vi "Process.vi"(8 "error in":errorcluster, 11 "Inst.AH2500":refnum<class "Inst.AH2500.lvclass">) -> (0 "error out":errorcluster, 3 "Inst.AH2500 out":refnum<class "Inst.AH2500.lvclass">)   [LabVIEW 2019, in "Inst.AH2500.lvclass"]
doc: "---------------------------------------------------------------\nJKI State Machine Objects™\nhttp://jki.net/state-machine-objects/\nCopyright (C) 2005-2015, JKI <info@jki.net>\nALL RIGHTS RESERVED"
uses:
  Inst.AH2500.lvclass
  <vilib>/JKI/JKI SMO/SMO/SMO.lvclass
  <userlib>/LevyLab/Instrument Framework/Instrument/Instrument.lvclass
  <userlib>/LevyLab/RemoteControl/RemoteControl/Typedefs/Message--Cluster.ctl
  <userlib>/LevyLab/RemoteControl/RemoteControl/RemoteControl.lvclass
  Typedefs/PrivateEvents--Inst.AH2500.MessageToProcess.ctl
  C:/Program Files/National Instruments/LabVIEW 2019/user.lib/LevyLab/Instrument Framework/Instrument Types/CBridge/Instrument.CBridge.lvclass
  C:/Program Files/National Instruments/LabVIEW 2019/user.lib/LevyLab/Instrument Framework/Instrument/Instrument.lvclass
  C:/Program Files/National Instruments/LabVIEW 2019/vi.lib/JKI/JKI SMO/SMO/SMO.lvclass
  <userlib>/LevyLab/Instrument Framework/Instrument/API/Instrument.sendMessageToProcess (variant).vi
  <userlib>/LevyLab/Debug/Debug.lvlib
  <userlib>/LevyLab/Instrument Framework/Instrument Types/CBridge/Instrument.CBridge.lvclass
panel:
  out "Status":string
  out "State History":string
  # "Inst.AH2500"
  # "Inst.AH2500"
  # "For instructions on how to use the JKI State Machine Objects, examples and video tutorials, visit:\nhttp://jki.net/state-machine-objects/\n\nJKI State Machine Objects™\nhttp://jki.net/state-machine-objects/\nCopyright (C) 2005-2015, JKI <info@jki.net>\nALL RIGHTS RESERVED"
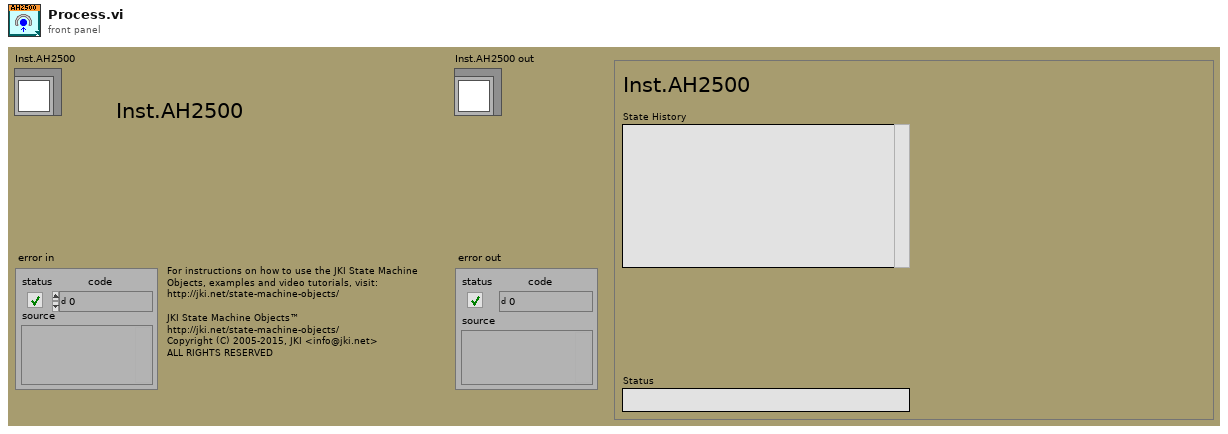
[diagram p1: front panel]
types:
  T1 = enum32{"invalid app kind", "Development System", "Run Time System", "Student Edition", "Embedded LabVIEW", "Evaluation", "Custom"}
  T2 = enum32{"Invalid", "Standard", "Closed", "Hidden", "Minimized", "Maximized"}
  T3 = typedef "RemoteControl.lvlib/RemoteControl.lvclass/Message--Cluster.ctl" = cluster{"Command":string, "Data":variant, "ID":string, "error":errorcluster}
  T4 = typedef "Inst.AH2500.lvclass/PrivateEvents--Inst.AH2500.MessageToProcess.ctl" = cluster{"Message":T3}
  T5 = cluster{"Core":cluster{"Current VI Reference":refnum<vi>, "Close Panel on Exit?":bool, "Last Error":cluster{"error":errorcluster, "previous state":string, "remaining states":string}, "Shutdown?":bool}, "SMO":refnum<class "Inst.AH2500.lvclass">, "Running Step":i32, "sequence":string[], "MessageToProcess":T4}
  T6 = cluster{"Current VI Reference":refnum<vi>, "Close Panel on Exit?":bool, "Last Error":cluster{"error":errorcluster, "previous state":string, "remaining states":string}, "Shutdown?":bool}
  T7 = typedef "Debug.lvlib/Attribute.Debug.lvclass/DebugBehavior.ctl" = enum16{"Normal", "Debug"}
  T8 = typedef "SMO.lvclass/Protected Events.ctl" = cluster{"StopProcesses":refnum<user-event>, "AbortProcesses":refnum<user-event>, "Config Changed":refnum<user-event>, "Dependency":refnum<user-event>}
  T9 = typedef "Inst.AH2500.lvclass/Inst.AH2500.getAll--Cluster.ctl" = cluster{"capacitance (pF)":dbl, "loss (nS)":dbl, "Vexc (V)":dbl}
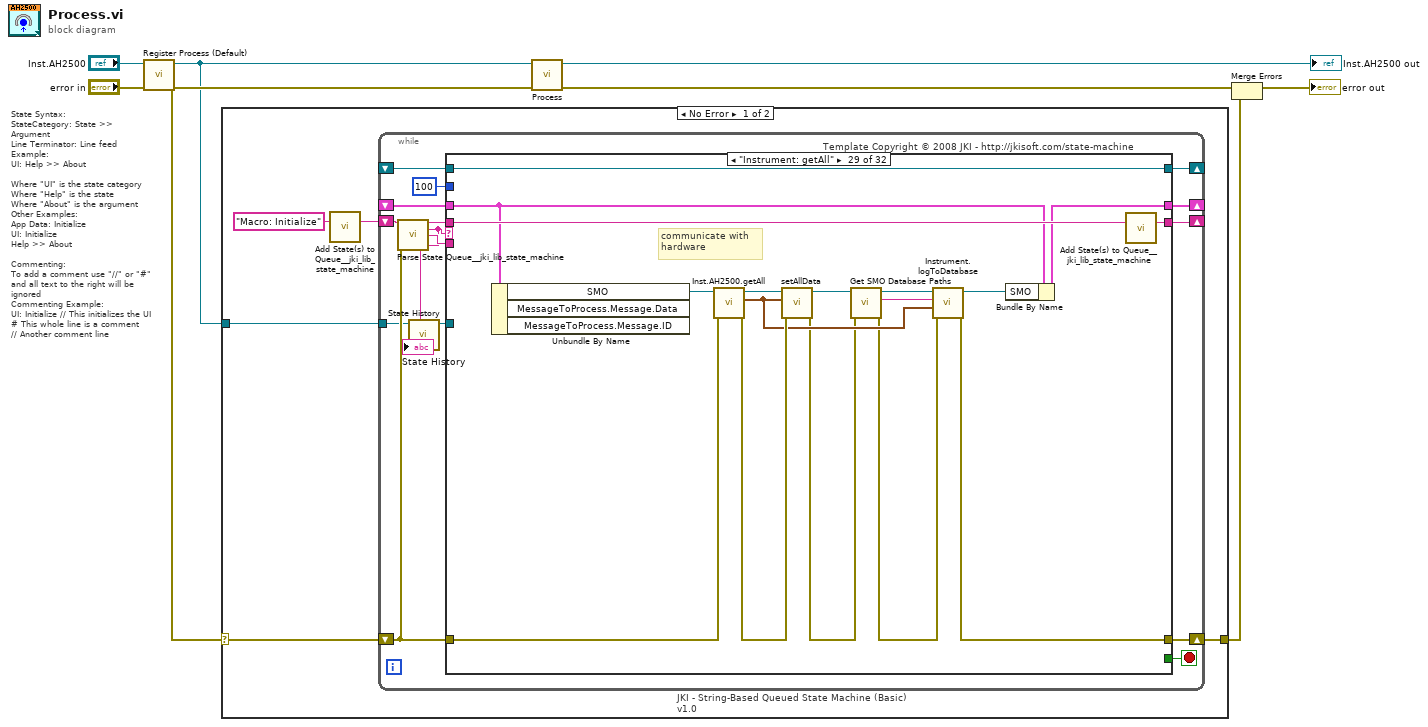
[diagram p0: block diagram]
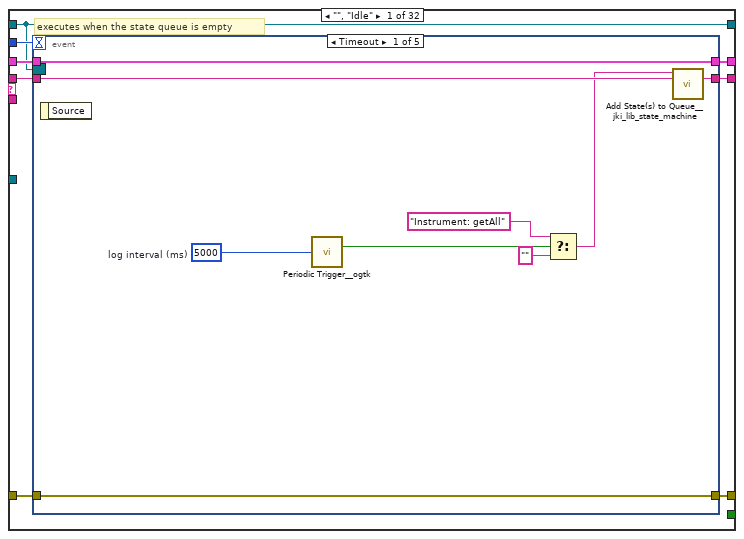
[diagram p2: hidden frame]
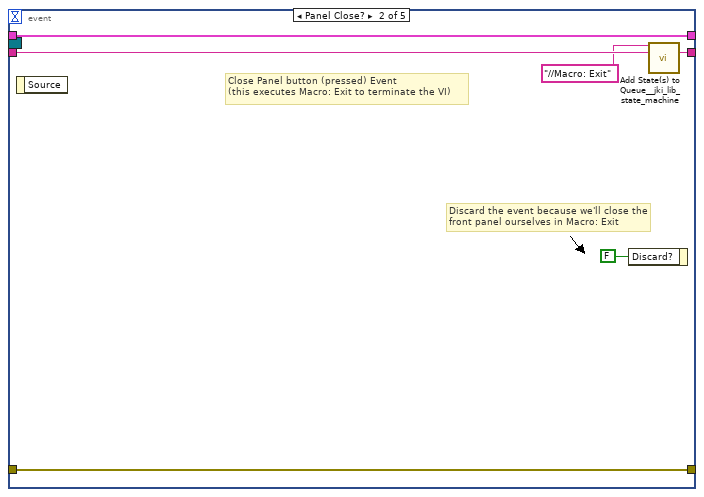
[diagram p3: hidden frame]
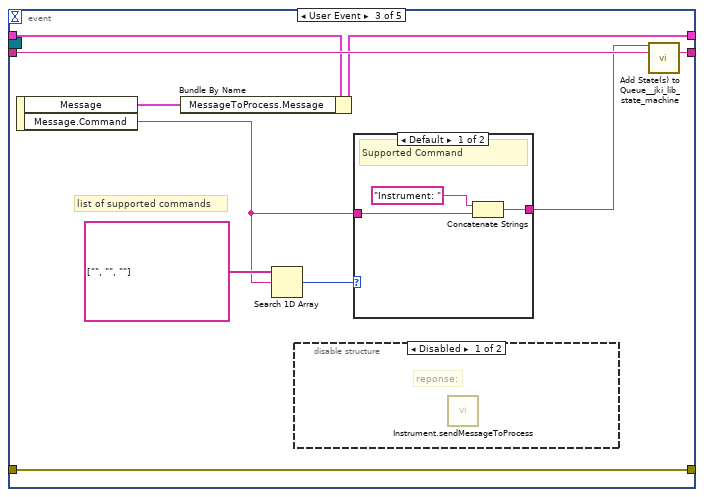
[diagram p4: hidden frame]
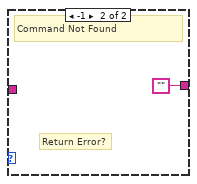
[diagram p6: hidden frame]
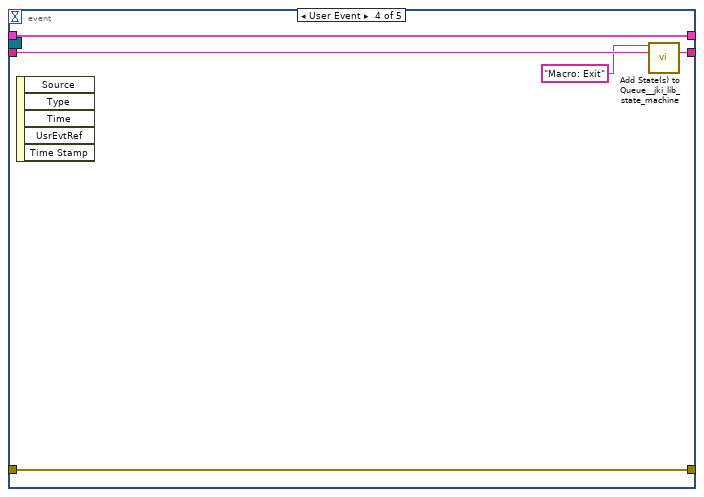
[diagram p7: hidden frame]
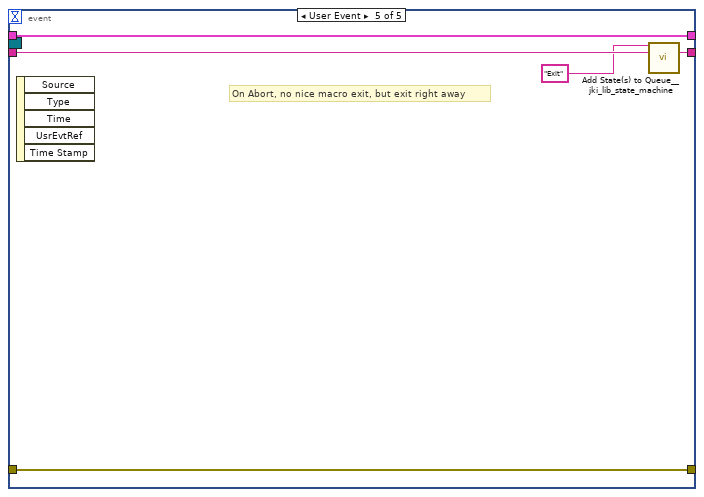
[diagram p8: hidden frame]
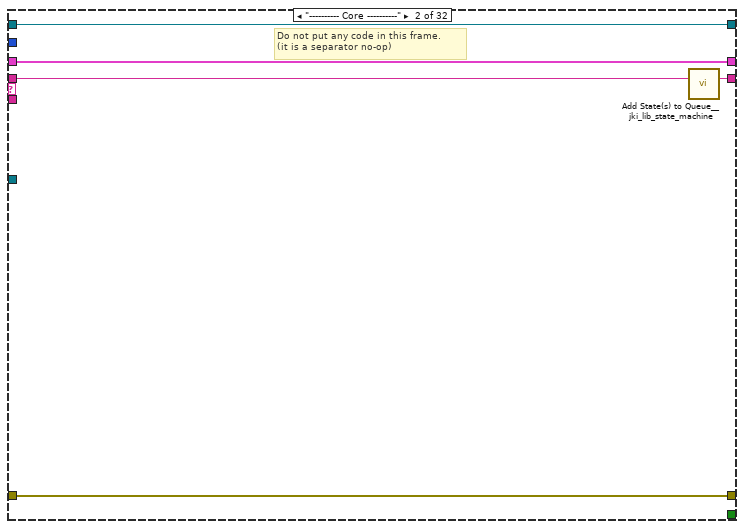
[diagram p9: hidden frame]
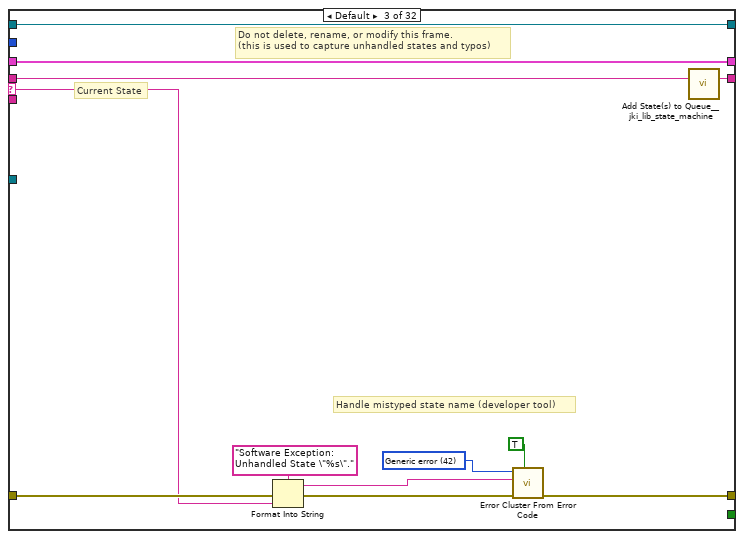
[diagram p10: hidden frame]
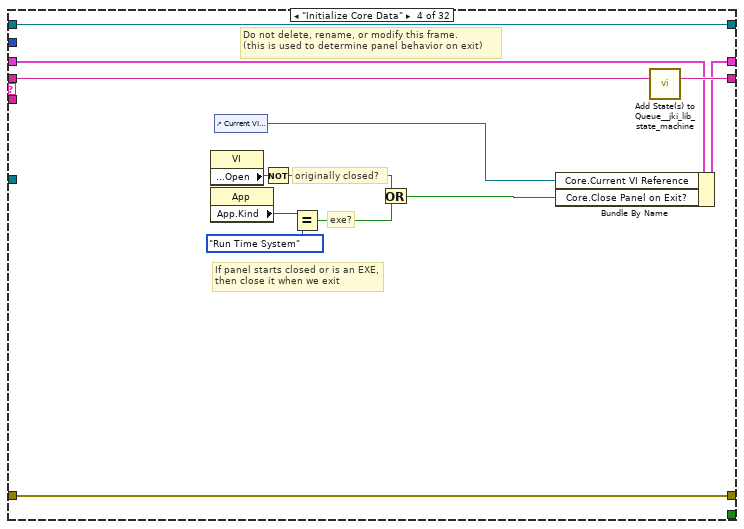
[diagram p11: hidden frame]
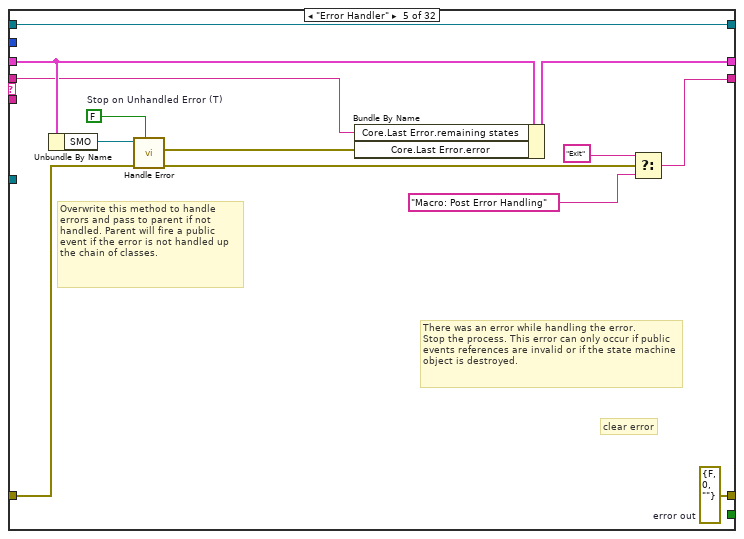
[diagram p12: hidden frame]
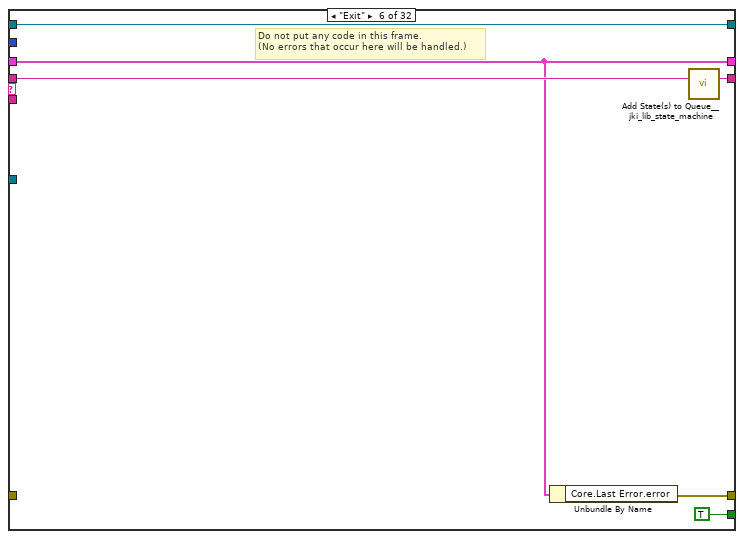
[diagram p13: hidden frame]
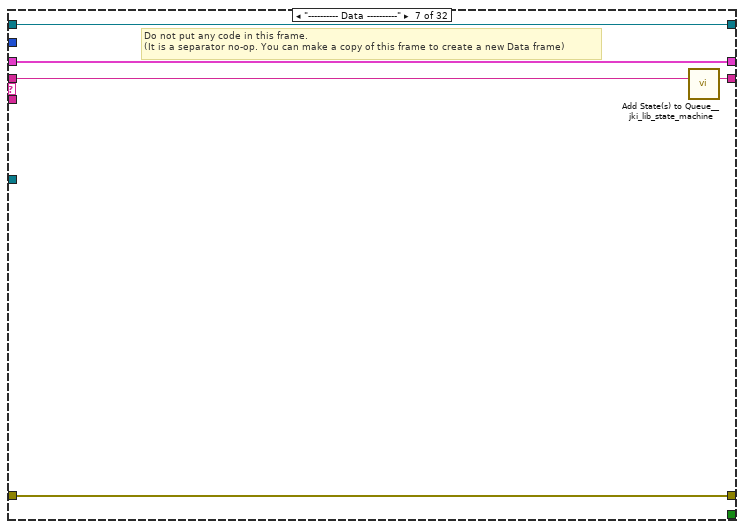
[diagram p14: hidden frame]
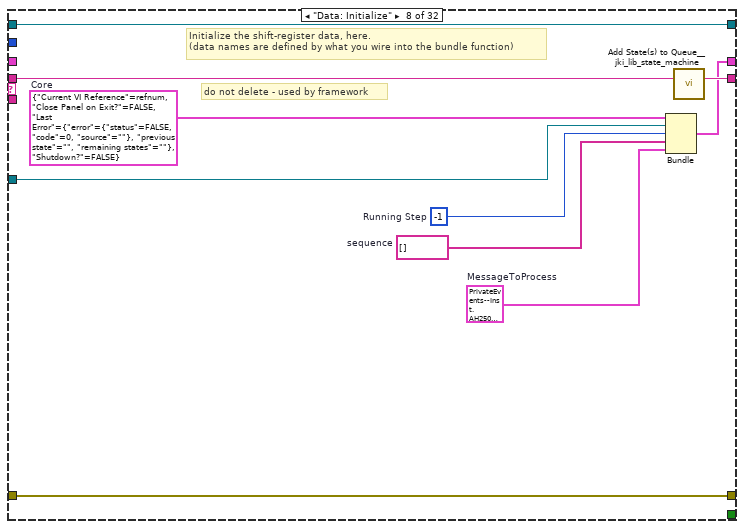
[diagram p15: hidden frame]
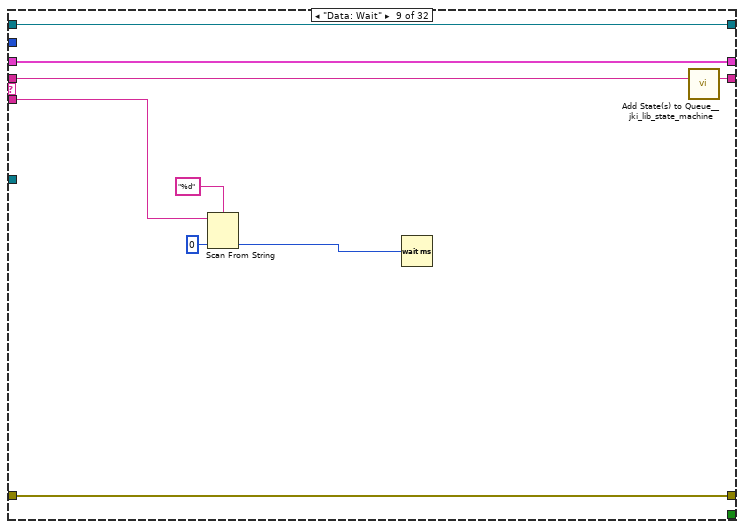
[diagram p16: hidden frame]
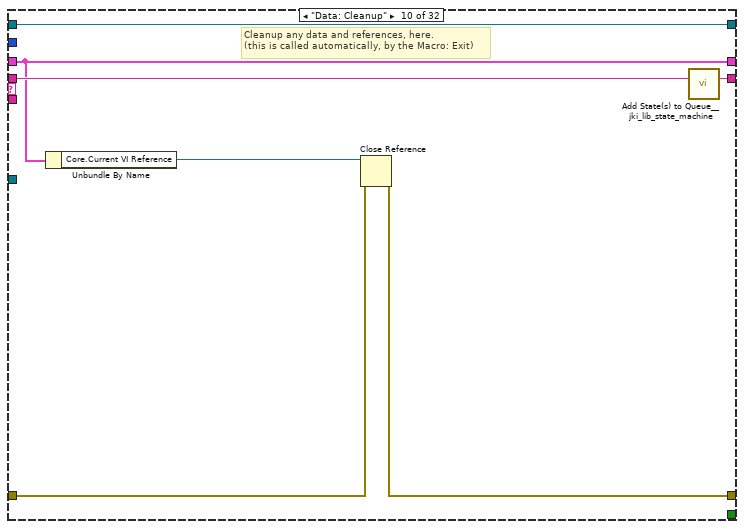
[diagram p17: hidden frame]
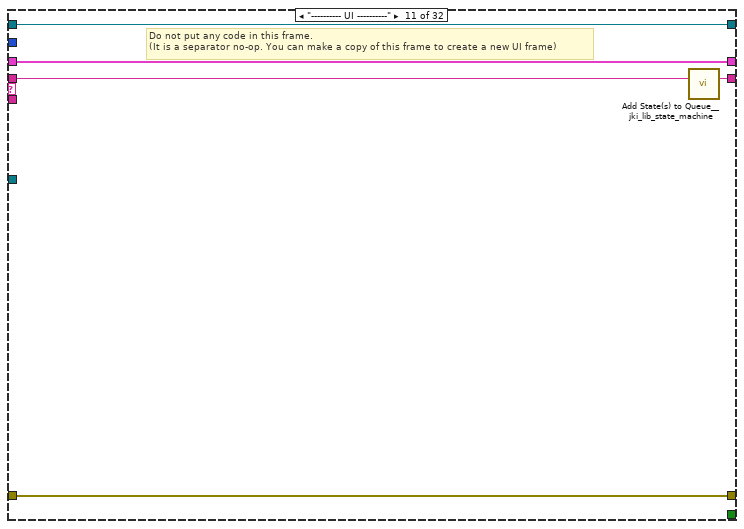
[diagram p18: hidden frame]
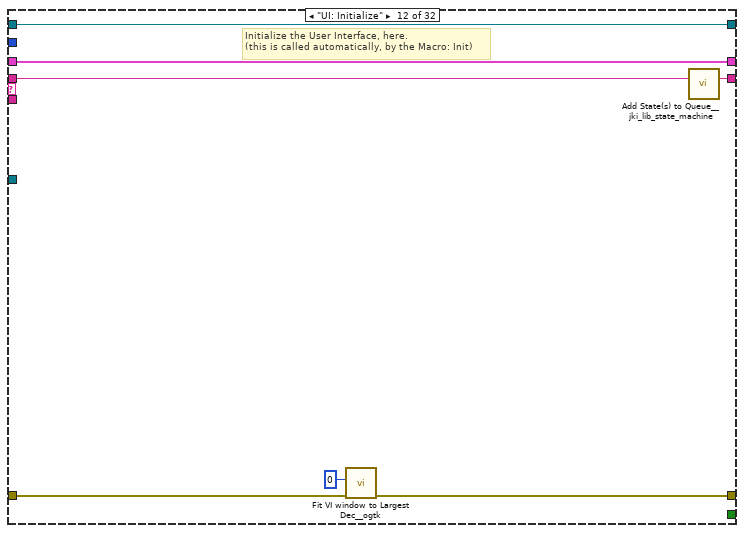
[diagram p19: hidden frame]
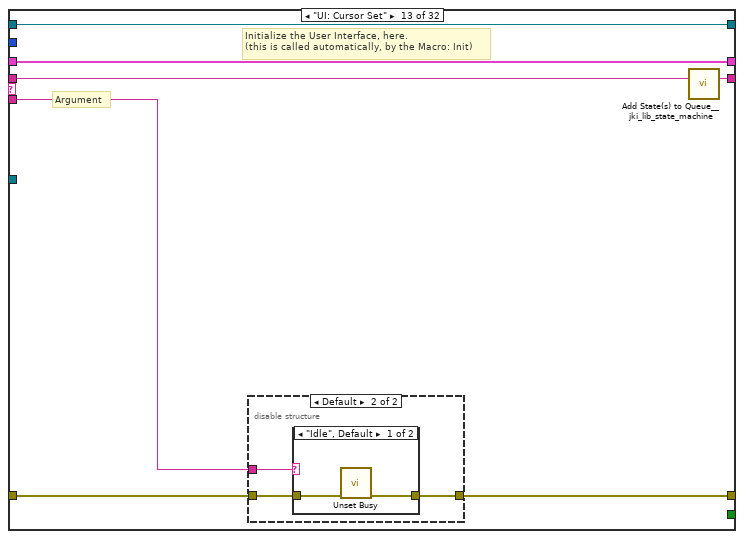
[diagram p20: hidden frame]
diagram:
  # "State Syntax:\nStateCategory: State >> Argument\nLine Terminator: Line feed\nExample:\nUI: Help >> About\n\nWhere \"UI\" is the state category\nWhere \"Help\" is the state\nWhere \"About\" is the argument\nOther Examples:\nApp Data: Initialize\nUI: Initialize\nHelp >> About\n\nCommenting:\nTo add a comment use \"//\" or \"#\" and all text to the right will be ignored\nCommenting Example:\nUI: Initialize // This initializes the UI\n# This whole line is a comment\n// Another comment line"
  n1 = call <vilib>:"Register Process (Default).vi"("error in (no error)"="error in", "SMO"="Inst.AH2500") -> ("error out"=w5:errorcluster, "SelfRef"=w4:refnum<class "Inst.AH2500.lvclass">)  [unwired: 8 in]
  n2 = case shown="No Error" w5 {
    selector: w5 -> [w10 w416]
    tunnel: w4 -> [w11 _]
    tunnel: [w9 w416] -> w1
    frame No Error {
      n3 = call <vilib>:"Add State(s) to Queue__jki_lib_state_machine.vi"("State(s) in (\"\")"="Macro: Initialize") -> ("States Out"=w13:string)  [unwired: 14 in]
      n4 = while "JKI - String-Based Queued State Machine (Basic) v1.0" {
        shift-right: [w23] -> _
        shift-left: _ -> [w22]
        shift-right: [w26] -> w9
        shift-left: w10 -> [w20]
        shift-right: [w25] -> _
        shift-left: w13 -> [w27]
        tunnel: w11 -> [w14]
        shift-right: [w19] -> _
        shift-left: _ -> [w18]
        stop <- w24 stop-if-true
        # "Template Copyright © 2008 JKI - http://jkisoft.com/state-machine"
        n5 = call <vilib>:"Parse State Queue__jki_lib_state_machine.vi"("State Queue"=w27, "Error In (no error)"=w20) -> ("Remaining States"=w29:string, "Current State"=w17:string, "Arguments"=w28:string)  [unwired: 11 in]
        n6 = call <userlib>:"State History.vi"("Current State"=w17, "SMO"=w14) -> ("SMO"=w15:refnum<class "Inst.AH2500.lvclass">, "History"=→"State History":string)  [unwired: 8 in]
        n7 = case shown="\"Instrument: getAll\"" w17 {
          selector: w17 -> [_ _ w83 _ _ _ _ _ _ _ _ _ _ _ _ _ _ _ _ _ _ _ _ _ _ _ _ _ _ _ _ _]
          tunnel: w29 -> [w37 w81 w87 w106 w111 w125 w130 w140 w149 w156 w161 w168 w175 w191 w223 w232 w236 w265 w286 w303 w308 w319 w324 w337 w343 w350 w359 w368 w385 w390 w396 w415]
          tunnel: w28 -> [_ _ _ _ _ _ _ _ w141 _ _ _ w169 w185 _ _ _ _ _ _ _ _ _ _ _ _ _ _ _ _ w391 w399]
          tunnel: w22 -> [w35 w78 w85 w97 w115 w121 w127 _ w146 w151 w158 w166 w173 w187 w220 w229 w235 w255 w276 w289 w305 w316 w321 w330 w341 w345 w355 w364 w381 w386 w392 w405]
          tunnel: [w34 w79 w89 w103 w116 w120 w128 w132 w147 w152 w159 w163 w170 w188 w221 w224 w239 w263 w284 w287 w306 w310 w322 w333 w339 w347 w352 w361 w369 w387 w393 w407] -> w26
          tunnel: w20 -> [w33 w79 w88 w103 w117 _ w128 w132 w147 w153 w159 w162 w171 w189 w221 w224 w238 w263 w284 w287 w306 w311 w322 w327 w339 w347 w351 w360 w379 w387 w393 w401]
          tunnel: [w36 w80 w86 w105 w107 w124 w129 w139 w148 w155 w160 w167 w174 w190 w222 w231 w234 w264 w285 w302 w307 w318 w323 w336 w342 w349 w358 w367 w384 w389 w395 w414] -> w25
          tunnel: [_ _ _ _ _ TRUE _ _ _ _ _ _ _ _ _ _ _ _ _ _ _ _ _ _ _ _ _ _ _ _ _ _] -> w24
          tunnel: [w32 w78 w85 w104 w114 w121 w127 w138 w146 w151 w158 w166 w173 w187 w220 w229 w237 w256 w277 w290 w305 w316 w321 w330 w341 w346 w356 w365 w382 w386 w392 w404] -> w23
          tunnel: 100 ("Timeout") -> [w31 _ _ _ _ _ _ _ _ _ _ _ _ _ _ _ _ _ _ _ _ _ _ _ _ _ _ _ _ _ _ _]
          tunnel: w15 -> [_ _ _ _ _ _ _ w133 _ _ _ _ _ _ _ _ _ _ _ _ _ _ _ _ _ _ _ _ _ _ _ _]
          tunnel: [w30 w77 w82 w94 w119 w122 w126 w137 w145 w150 w157 w165 w172 w184 w219 w230 w247 w262 w283 w297 w304 w317 w320 w335 w340 w348 w357 w366 w383 w388 w394 w413] -> w19
          tunnel: w18 -> [w30 w77 w82 w94 w119 w122 w126 w137 w145 w150 w157 w165 w172 w184 w219 w230 w247 w262 w283 w297 w304 w317 w320 _ w340 w348 w357 w366 w383 w388 w394 w413]
          frame "", "Idle" {
            # "executes when the state queue is empty"
            n8 = event shown="[0] Timeout" {
              selector: w30 -> [_ _ _ _ _]
              dyn-events: _ -> [_ _ _ _ _]
              timeout: w31 -> [_ _ _ _ _]
              tunnel: w37 -> [w46 w52 w62 w71 w76]
              tunnel: [w45 w51 w61 w70 w75] -> w36
              tunnel: w35 -> [w43 w49 w54 w68 w73]
              tunnel: [w44 w50 w60 w69 w74] -> w34
              tunnel: w33 -> [w44 w50 w60 w69 w74]
              tunnel: [w43 w49 w55 w68 w73] -> w32
              event Timeout {
                w40 = u32 5000  # log interval (ms)
                n9 = event-data() -> ()  [unwired: 1 in, 1 out]
                n10 = call <userlib>:"Periodic Trigger__ogtk.vi"("time (ms)"=w40) -> ("Triggered"=w42:bool)  [unwired: 12 in, 2 out]
                n11 = Select(t="Instrument: getAll", s=w42, f="") -> (s? t:f=w39:string)
                n12 = call <vilib>:"Add State(s) to Queue__jki_lib_state_machine.vi"("State(s) in Front (\"\")"=w39, "State(s) in (\"\")"=w46) -> ("States Out"=w45:string)  [unwired: 13 in]
              }
              event Panel Close? {
                # "Discard the event because we'll close the front panel ourselves in Macro: Exit"
                # "Close Panel button (pressed) Event\n(this executes Macro: Exit to terminate the VI)"
                n13 = event-data() -> ()  [unwired: 1 in, 1 out]
                n14 = event-data("Discard?"=FALSE) -> ()  [unwired: 1 in, 1 out]
                n15 = call <vilib>:"Add State(s) to Queue__jki_lib_state_machine.vi"("State(s) in Front (\"\")"="//Macro: Exit", "State(s) in (\"\")"=w52) -> ("States Out"=w51:string)  [unwired: 13 in]
              }
              event User Event {
                # "list of supported commands"
                n16 = event-data() -> ("Message"=w53:T3, "Message.Command"=w56:string)  [unwired: 1 in]
                n17 = Bundle By Name(cluster=w54, "MessageToProcess.Message"=w53) -> (w55:T5)
                n18 = Search 1D Array(1D array=string[] ["", "", ""], element=w56) -> (index of element=w59:i32)  [unwired: 1 in]
                n19 = disable-structure shown="Disabled" {
                  frame Disabled {
                    # "reponse:"
                    n20 = call-poly <userlib>:"Instrument.sendMessageToProcess.vi"() -> ()  [unwired: 10 in, 2 out]
                  }
                  frame Enabled {
                  }
                }
                n21 = case shown="Default" w59 {
                  tunnel: [w65 "" ("Empty String Constant")] -> w57
                  tunnel: w56 -> [w64 _]
                  frame Default {
                    # "Supported Command"
                    n22 = Concatenate Strings("Instrument: ", w64) -> (w65:string)
                  }
                  frame -1 {
                    # "Return Error?"
                    # "Command Not Found"
                  }
                }
                n23 = call <vilib>:"Add State(s) to Queue__jki_lib_state_machine.vi"("State(s) in Front (\"\")"=w57, "State(s) in (\"\")"=w62) -> ("States Out"=w61:string)  [unwired: 13 in]
              }
              event User Event {
                n24 = event-data() -> ()  [unwired: 1 in, 5 out]
                n25 = call <vilib>:"Add State(s) to Queue__jki_lib_state_machine.vi"("State(s) in Front (\"\")"="Macro: Exit", "State(s) in (\"\")"=w71) -> ("States Out"=w70:string)  [unwired: 13 in]
              }
              event User Event {
                # "On Abort, no nice macro exit, but exit right away"
                n26 = event-data() -> ()  [unwired: 1 in, 5 out]
                n27 = call <vilib>:"Add State(s) to Queue__jki_lib_state_machine.vi"("State(s) in Front (\"\")"="Exit", "State(s) in (\"\")"=w76) -> ("States Out"=w75:string)  [unwired: 13 in]
              }
            }
          }
          frame "---------- Core ----------" {
            # "Do not put any code in this frame.\n(it is a separator no-op)"
            n28 = call <vilib>:"Add State(s) to Queue__jki_lib_state_machine.vi"("State(s) in (\"\")"=w81) -> ("States Out"=w80:string)  [unwired: 14 in]
          }
          frame Default {
            w92 = 42 items=["No error", "Argument error", "Memory is full", "Out of zone", "End of file", "File already open", "Generic file I/O error", "File not found", "File permission error", "Disk is full", "Duplicate path", "Too many files open", "System feature not enabled", "Resource file not found", "Cannot add resource", "Resource not found", "Image not found", "Image memory error", "Pen does not exist", "Config type invalid", "Config token not found", "Config parse error", "Config memory error", "Bad external code format", "Bad external code offset", "External code not present", "Null window", "Destroy window error", "Null menu", "Print aborted", "Bad print record", "Print driver error", "Windows error during printing", "Memory error during printing", "Print dialog error", "Generic print error", "Invalid device refnum", "Device not found", "Device parameter error", "Device unit error", "Cannot open device", "Device call aborted", "Generic error", "Cancelled by user", "Object ID too low", "Object ID too high", "Object not in heap", "Unknown heap", "Unknown object (invalid DefProc)", "Unknown object (DefProc not in table)", "Message out of range", "Invalid (null) method", "Unknown message", "Manager call not supported", "Bad address", "Network operation in progress", "Network operation timed out", "Connection is busy", "Network attribute not supported", "Network error", "Address in use", "System out of memory", "Connection aborted", "Connection refused", "Not connected", "Already connected", "Connection closed", "Initialization error (interapplication manager)", "Bad occurrence", "Wait on unbound occurrence handler", "Occurrence queue overflow", "Datalog type conflict", "Unused", "Unrecognized type (interapplication manager)", "Memory corrupt", "Failed to make temporary DLL", "Old CIN version", "Drag socket not found", "Failed to load drop-object", "Failed to register OLE object", "Failed to release OLE object", "Format specifier type mismatch", "Unknown format specifier", "Too few format specifiers", "Too many format specifiers", "Scan failed", "Newer CIN version", "Error converting to variant", "Runtime menu error", "Password tampered", "Variant attribute not found", "Incompatible variant data type", "Event data is not available", "Event Store is not present", "Occurrence is not found", "Event Queue is not created", "Event info is not available", "Refnum passed is NULL", "Error retrieving Class GUID", "Error retrieving CoClass GUID", "Error retrieving TypeLib GUID.", "Bad built application magic bytes.", "Specific driver is different from the specific driver associated with the Logical Name.", "There is no session opened to the class driver.", "Max Error", "MAX - Error with config objects", "MAX - Error loading configuration", "MAX - Group not supported"]
            # "Current State"
            # "Do not delete, rename, or modify this frame.\n(this is used to capture unhandled states and typos)"
            # "Handle mistyped state name (developer tool)"
            n29 = Format Into String(format string="Software Exception: Unhandled State \"%s\"." ("message"), error in=w88, w83) -> (resulting string=w91:string, error out=w90:errorcluster)  [unwired: 1 in]
            n30 = call <vilib>:"Error Cluster From Error Code.vi"("show call chain? (False)"=TRUE, "error in (no error)"=w90, "error message (\"\")"=w91, "error code (0)"=w92) -> ("error out"=w89:errorcluster)  [unwired: 5 in]
            n31 = call <vilib>:"Add State(s) to Queue__jki_lib_state_machine.vi"("State(s) in (\"\")"=w87) -> ("States Out"=w86:string)  [unwired: 14 in]
          }
          frame "Initialize Core Data" {
            # "Do not delete, rename, or modify this frame.\n(this is used to determine panel behavior on exit)"
            # "originally closed?"
            # "exe?"
            # "If panel starts closed or is an EXE, then close it when we exit"
            n32 = property class="VI"() -> ("Front Panel.Open"=w102:bool)  [unwired: 2 in, 2 out]
            n33 = property class="App"() -> ("App.Kind"=w101:T1)  [unwired: 2 in, 2 out]
            n34 = control-ref of="Current VI Reference"() -> (w95:refnum<vi>)
            n35 = Not(x=w102) -> (.not. x?=w99:bool)
            n36 = Equal?(x=w101, y=T1."Run Time System" ("Application:Kind")) -> (x = y?=w98:bool)
            n37 = Or(x=w99, y=w98) -> (x .or. y?=w96:bool)
            n38 = Bundle By Name(cluster=w97, "Core.Current VI Reference"=w95, "Core.Close Panel on Exit?"=w96) -> (w104:T5)
            n39 = call <vilib>:"Add State(s) to Queue__jki_lib_state_machine.vi"("State(s) in (\"\")"=w106) -> ("States Out"=w105:string)  [unwired: 14 in]
          }
          frame "Error Handler" {
            w112 = FALSE  # Stop on Unhandled Error (T)
            w116 = errorcluster {"status"=FALSE, "code"=0, "source"=""}  # error out
            # "clear error"
            # "There was an error while handling the error.\nStop the process. This error can only occur if public events references are invalid or if the state machine object is destroyed."
            # "Overwrite this method to handle errors and pass to parent if not handled. Parent will fire a public event if the error is not handled up the chain of classes."
            n40 = Unbundle By Name(w115) -> ("SMO"=w118:refnum<class "Inst.AH2500.lvclass">)
            n41 = call-dynamic "Handle Error.vi"("Stop on Unhandled Error (T)"=w112, "error in"=w117, "SMO"=w118) -> ("handling error"=w108:errorcluster, "Unhandled error"=w113:errorcluster)  [unwired: 6 in, 1 out]
            n42 = Bundle By Name(cluster=w115, "Core.Last Error.remaining states"=w111, "Core.Last Error.error"=w113) -> (w114:T5)
            n43 = Select(t="Exit", s=w108, f="Macro: Post Error Handling") -> (s? t:f=w107:string)
          }
          frame "Exit" {
            # "Do not put any code in this frame.\n(No errors that occur here will be handled.)"
            n44 = Unbundle By Name(w121) -> ("Core.Last Error.error"=w120:errorcluster)
            n45 = call <vilib>:"Add State(s) to Queue__jki_lib_state_machine.vi"("State(s) in (\"\")"=w125) -> ("States Out"=w124:string)  [unwired: 14 in]
          }
          frame "---------- Data ----------" {
            # "Do not put any code in this frame.\n(It is a separator no-op. You can make a copy of this frame to create a new Data frame)"
            n46 = call <vilib>:"Add State(s) to Queue__jki_lib_state_machine.vi"("State(s) in (\"\")"=w130) -> ("States Out"=w129:string)  [unwired: 14 in]
          }
          frame "Data: Initialize" {
            w131 = T4 {"Message"={"Command"="", "Data"=variant(string ""), "ID"="", "error"={"status"=FALSE, "code"=0, "source"=""}}}  # MessageToProcess
            w134 = string[] []  # sequence
            w135 = -1  # Running Step
            w136 = T6 {"Current VI Reference"=refnum, "Close Panel on Exit?"=FALSE, "Last Error"={"error"={"status"=FALSE, "code"=0, "source"=""}, "previous state"="", "remaining states"=""}, "Shutdown?"=FALSE}  # Core
            # "do not delete - used by framework"
            # "Initialize the shift-register data, here.\n(data names are defined by what you wire into the bundle function)"
            n47 = Bundle("Core"=w136, "SMO"=w133, "Running Step"=w135, "sequence"=w134, "MessageToProcess"=w131) -> (w138:T5)  [unwired: 1 in]
            n48 = call <vilib>:"Add State(s) to Queue__jki_lib_state_machine.vi"("State(s) in (\"\")"=w140) -> ("States Out"=w139:string)  [unwired: 14 in]
          }
          frame "Data: Wait" {
            n49 = Scan From String(format string="%d", input string=w141, default 1=u32 0 ("default value 1")) -> (output 1=w142:u32)  [unwired: 2 in, 3 out]
            n50 = Wait (ms)(milliseconds to wait=w142) -> ()  [unwired: 1 out]
            n51 = call <vilib>:"Add State(s) to Queue__jki_lib_state_machine.vi"("State(s) in (\"\")"=w149) -> ("States Out"=w148:string)  [unwired: 14 in]
          }
          frame "Data: Cleanup" {
            # "Cleanup any data and references, here.\n(this is called automatically, by the Macro: Exit)"
            n52 = Unbundle By Name(w151) -> ("Core.Current VI Reference"=w154:refnum<vi>)
            n53 = Close Reference(reference=w154, error in (no error)=w153) -> (error out=w152:errorcluster)
            n54 = call <vilib>:"Add State(s) to Queue__jki_lib_state_machine.vi"("State(s) in (\"\")"=w156) -> ("States Out"=w155:string)  [unwired: 14 in]
          }
          frame "---------- UI ----------" {
            # "Do not put any code in this frame.\n(It is a separator no-op. You can make a copy of this frame to create a new UI frame)"
            n55 = call <vilib>:"Add State(s) to Queue__jki_lib_state_machine.vi"("State(s) in (\"\")"=w161) -> ("States Out"=w160:string)  [unwired: 14 in]
          }
          frame "UI: Initialize" {
            # "Initialize the User Interface, here.\n(this is called automatically, by the Macro: Init)"
            n56 = call <userlib>:"Fit VI window to Largest Dec__ogtk.vi"("error in (no error)"=w162, "border spacing (2 px)"=0) -> ("error out"=w163:errorcluster)  [unwired: 4 in, 1 out]
            n57 = call <vilib>:"Add State(s) to Queue__jki_lib_state_machine.vi"("State(s) in (\"\")"=w168) -> ("States Out"=w167:string)  [unwired: 14 in]
          }
          frame "UI: Cursor Set" {
            # "Argument"
            # "Initialize the User Interface, here.\n(this is called automatically, by the Macro: Init)"
            n58 = disable-structure shown="Default" {
              disable-tunnel: w171 -> [w176 w179]
              disable-tunnel: [w176 w178] -> w170
              disable-tunnel: w169 -> [_ w177]
              frame condition #0 {
              }
              frame condition #1 (active) {
                n59 = case shown="\"Idle\", Default" w177 {
                  tunnel: w179 -> [w181 w183]
                  tunnel: [w180 w182] -> w178
                  frame "Idle", Default {
                    n60 = call <vilib>:"Unset Busy.vi"("error in (no error)"=w181) -> ("error out"=w180:errorcluster)  [unwired: 10 in]
                  }
                  frame "Busy" {
                    n61 = call <vilib>:"Set Busy.vi"("error in (no error)"=w183) -> ("error out"=w182:errorcluster)  [unwired: 9 in, 1 out]
                  }
                }
              }
            }
            n62 = call <vilib>:"Add State(s) to Queue__jki_lib_state_machine.vi"("State(s) in (\"\")"=w175) -> ("States Out"=w174:string)  [unwired: 14 in]
          }
          frame "UI: Front Panel State" {
            # "Argument"
            # "Set Front Panel Open or Closed\n(Usage: \"UI: Front Panel State >> Open|Close\")"
            n63 = Unbundle By Name(w187) -> ("Core.Current VI Reference"=w186:refnum<vi>)
            n64 = disable-structure shown="TARGET_TYPE==RT" {
              disable-tunnel: w189 -> [w195 w218]
              disable-tunnel: [w194 w218] -> w188
              disable-tunnel: w186 -> [w193 _]
              disable-tunnel: w185 -> [w192 _]
              frame condition #0 (active) {
                n65 = case shown="\"Close\"" w192 {
                  tunnel: w195 -> [w199 w212]
                  tunnel: [w201 w213] -> w194
                  tunnel: w193 -> [w200 w210]
                  frame "Open", Default {
                    n66 = property class="VI"(reference=w200, error in=w199) -> (reference out=w197:refnum<vi>, error out=w198:errorcluster, "FP.State"=w196:T2)
                    n67 = case shown="\"Closed\"" w196 {
                      tunnel: [w204 w207] -> w201
                      tunnel: w198 -> [w203 w207]
                      tunnel: w197 -> [w202 _]
                      frame "Closed" {
                        n68 = invoke class="VI" method="FP.Open"(reference=w202, error in=w203, "Activate"=TRUE, "State"=T2."Standard") -> (error out=w204:errorcluster)  [unwired: 1 in, 4 out]
                      }
                      frame Default {
                      }
                    }
                  }
                  frame "Close" {
                    n69 = property class="VI"(reference=w210, error in=w212) -> (reference out=w209:refnum<vi>, error out=w211:errorcluster, "FP.State"=w208:T2)
                    n70 = case shown="Default" w208 {
                      tunnel: [w214 w217] -> w213
                      tunnel: w211 -> [w214 w216]
                      tunnel: w209 -> [_ w215]
                      frame "Invalid", "Closed" {
                      }
                      frame Default {
                        n71 = invoke class="VI" method="FP.Close"(reference=w215, error in=w216) -> (error out=w217:errorcluster)  [unwired: 1 in, 2 out]
                      }
                    }
                  }
                }
              }
              frame condition #1 {
              }
            }
            n72 = call <vilib>:"Add State(s) to Queue__jki_lib_state_machine.vi"("State(s) in (\"\")"=w191) -> ("States Out"=w190:string)  [unwired: 14 in]
          }
          frame "---------- Macro ----------" {
            # "Do not put any code in this frame.\n(It is a separator no-op. You can make a copy of this frame to create a new Macro frame)"
            n73 = call <vilib>:"Add State(s) to Queue__jki_lib_state_machine.vi"("State(s) in (\"\")"=w223) -> ("States Out"=w222:string)  [unwired: 14 in]
          }
          frame "Macro: Initialize" {
            # "Initialization Macro\n(This is called once, when the VI starts)"
            n74 = call <vilib>:"Add State(s) to Queue__jki_lib_state_machine.vi"("State(s) in Front (\"\")"="Data: Initialize\nInitialize Core Data\nEvents: Register", "State(s) in (\"\")"="Process: Sync", "State(s) at Back (\"\")"="UI: Initialize\nUI: Front Panel State >> Close\nMacro: Debug\nInstrument: Open Hardware\nInstrument: getAll") -> ("States Out"=w227:string)  [unwired: 12 in]
            n75 = call <vilib>:"Add State(s) to Queue__jki_lib_state_machine.vi"("State(s) in Front (\"\")"=w227, "State(s) in (\"\")"=w232) -> ("States Out"=w231:string)  [unwired: 13 in]
          }
          frame "Macro: Debug" {
            # "exe?"
            # "If pane is an EXE, then close it when we exit"
            # "Macro: Debug\n(get debug behavior, determine UI and determine shutdown behavior)"
            n76 = Unbundle By Name(w235) -> ("Core.Close Panel on Exit?"=w241:bool, "SMO"=w246:refnum<class "Inst.AH2500.lvclass">)
            n77 = property class="App"() -> ("App.Kind"=w244:T1)  [unwired: 2 in, 2 out]
            n78 = Equal?(x=w244, y=T1."Run Time System" ("Application:Kind")) -> (x = y?=w240:bool)
            n79 = call <userlib>:"Get Debug Mode.vi"("error in (no error)"=w238, "SMO"=w246) -> ("error out"=w239:errorcluster, "Behavior"=w245:T7)  [unwired: 7 in, 1 out]
            n80 = case shown="\"Debug\"" w245 {
              tunnel: [w249 w251] -> w242
              tunnel: w241 -> [w249 _]
              tunnel: w240 -> [_ w253]
              tunnel: ["" "UI: Front Panel State >> Open\nUI: Wait >> 1000"] -> w233
              frame "Normal", Default {
                # "respect core.close"
              }
              frame "Debug" {
                # "keep panel open\nunless exe"
                n81 = Or(x=w253, y=FALSE) -> (x .or. y?=w251:bool)
              }
            }
            n82 = Bundle By Name(cluster=w235, "Core.Close Panel on Exit?"=w242) -> (w237:T5)
            n83 = call <vilib>:"Add State(s) to Queue__jki_lib_state_machine.vi"("State(s) in Front (\"\")"=w233, "State(s) in (\"\")"=w236) -> ("States Out"=w234:string)  [unwired: 13 in]
          }
          frame "Macro: Post Error Handling" {
            # "Clear Last Error?"
            n84 = Unbundle By Name(w255) -> ("Core.Last Error.remaining states"=w257:string, "Core.Shutdown?"=w258:bool)
            n85 = Unbundle By Name(w255) -> ("Core.Last Error.error"=w261:errorcluster)
            n86 = case shown="False" FALSE {
              tunnel: w261 -> [w269 _]
              tunnel: [w269 _] -> w260
              frame False {
              }
              frame True {
              }
            }
            n87 = case shown="True" w258 {
              tunnel: w257 -> [w266 w268]
              tunnel: [w266 w267] -> w254
              frame False {
                # "These are the remaining states (at the moment the error occured). States can be altered according to business logic."
                # "NOT SHUTTING DOWN"
              }
              frame True {
                # "Developer can decide to alter the states but should be aware that during the shutdown process, there are certain states that must be run for the SMO to properly shut itself (and this process) down. As such, one can add states to perform additional clean-ups, but should append the remaining state to be executed."
                # "SHUTTING DOWN"
                n88 = call <vilib>:"Add State(s) to Queue__jki_lib_state_machine.vi"("State(s) in (\"\")"=w268) -> ("States Out"=w267:string)  [unwired: 14 in]
              }
            }
            n89 = Bundle By Name(cluster=w255, "Core.Last Error.error"=w260) -> (w256:T5)
            n90 = call <vilib>:"Add State(s) to Queue__jki_lib_state_machine.vi"("State(s) in Front (\"\")"=w254, "State(s) in (\"\")"=w265) -> ("States Out"=w264:string)  [unwired: 13 in]
          }
          frame "Macro: Run Sequence" {
            # "0,1,2,3,4,"
            # "5"
            # "Do not put any code in this frame.\n(It is a separator no-op. You can make a copy of this frame to create a new Macro frame)"
            n91 = Unbundle By Name(w276) -> ("sequence"=w272:string[], "Running Step"=w270:i32)
            n92 = Array Size(array=w272) -> (size(s)=w282:i32)
            n93 = Index Array(array=w272, index=w270) -> (element=w271:string)
            n94 = Greater Or Equal?(x=w282, y=w270) -> (x >= y?=w274:bool)
            n95 = Select(t=-1 ("Running Step"), s=w274, f=w270) -> (s? t:f=w281:i32)
            n96 = Bundle By Name(cluster=w276, "Running Step"=w281) -> (w277:T5)
            n97 = Select(t="Sequence: Status >> ...", s=w274, f="Idle //Check Event Structure\nMacro: Run Sequence" ("State(s) at Back (\"\")")) -> (s? t:f=w273:string)
            n98 = call <vilib>:"Add State(s) to Queue__jki_lib_state_machine.vi"("State(s) in Front (\"\")"=w271, "State(s) at Back (\"\")"=w273) -> ("States Out"=w275:string)  [unwired: 13 in]
            n99 = call <vilib>:"Add State(s) to Queue__jki_lib_state_machine.vi"("State(s) in Front (\"\")"=w275, "State(s) in (\"\")"=w286) -> ("States Out"=w285:string)  [unwired: 13 in]
          }
          frame "Macro: Exit" {
            # "Exit Macro\n(This is called once, when the VI exits)"
            n100 = Unbundle By Name(w289) -> ("Core.Close Panel on Exit?"=w301:bool)
            n101 = Bundle By Name(cluster=w289, "Core.Shutdown?"=TRUE) -> (w290:T5)
            n102 = Select(t="UI: Front Panel State >> Close", s=w301, f="" ("Empty String Constant")) -> (s? t:f=w299:string)
            n103 = call <vilib>:"Add State(s) to Queue__jki_lib_state_machine.vi"("State(s) in Front (\"\")"="Data: Cleanup\nEvents: Unregister", "State(s) in (\"\")"="Process: Sync", "State(s) at Back (\"\")"="Exit") -> ("States Out"=w294:string)  [unwired: 12 in]
            n104 = call <vilib>:"Add State(s) to Queue__jki_lib_state_machine.vi"("State(s) in Front (\"\")"="Instrument: Close Hardware", "State(s) in (\"\")"=w299, "State(s) at Back (\"\")"=w294) -> ("States Out"=w298:string)  [unwired: 12 in]
            n105 = call <vilib>:"Add State(s) to Queue__jki_lib_state_machine.vi"("State(s) in Front (\"\")"=w298, "State(s) in (\"\")"=w303) -> ("States Out"=w302:string)  [unwired: 13 in]
          }
          frame "---------- Process ----------" {
            # "Template Separator\n(You can make a copy of, or modify, this frame)"
            n106 = call <vilib>:"Add State(s) to Queue__jki_lib_state_machine.vi"("State(s) in (\"\")"=w308) -> ("States Out"=w307:string)  [unwired: 14 in]
          }
          frame "Process: Sync" {
            n107 = Unbundle By Name(w316) -> ("SMO"=w312:refnum<class "Inst.AH2500.lvclass">)
            n108 = call <vilib>:"WaitOnProcessSync.vi"("error in (no error)"=w311, "SMO"=w312) -> ("error out"=w310:errorcluster, "Don't run?"=w315:bool)  [unwired: 7 in, 1 out]
            n109 = Select(t="Data: Cleanup\nEvents: Unregister\nExit", s=w315, f="" ("Empty String Constant")) -> (s? t:f=w309:string)
            n110 = call <vilib>:"Add State(s) to Queue__jki_lib_state_machine.vi"("State(s) in Front (\"\")"=w309, "State(s) in (\"\")"=w319) -> ("States Out"=w318:string)  [unwired: 13 in]
          }
          frame "---------- Events ----------" {
            # "Template Separator\n(You can make a copy of, or modify, this frame)"
            n111 = call <vilib>:"Add State(s) to Queue__jki_lib_state_machine.vi"("State(s) in (\"\")"=w324) -> ("States Out"=w323:string)  [unwired: 14 in]
          }
          frame "Events: Register" {
            n112 = Unbundle By Name(w330) -> ("SMO"=w331:refnum<class "Inst.AH2500.lvclass">)
            n113 = call <vilib>:"GetProtectedEvents.vi"("SMO"=w331) -> ("error out"=w329:errorcluster, "SMO Protected Events"=w334:T8, "SMO out"=w328:refnum<class "Inst.AH2500.lvclass">)  [unwired: 8 in]
            n114 = call "Inst.AH2500.GetPrivateEvents.vi"("Inst.AH2500 in"=w328) -> ("error out"=w325:errorcluster, "Inst.AH2500 Private Events"=w326:cluster{"MessageToProcess":refnum<user-event>})  [unwired: 8 in, 1 out]
            n115 = register-events(w334, w326) -> (reference out=w335:refnum<event-registration>, error out=w332:errorcluster)  [unwired: 2 in]
            n116 = Merge Errors(w332, w325, w329, w327) -> (w333:errorcluster)
            n117 = call <vilib>:"Add State(s) to Queue__jki_lib_state_machine.vi"("State(s) in (\"\")"=w337) -> ("States Out"=w336:string)  [unwired: 14 in]
          }
          frame "Events: Unregister" {
            n118 = Unregister For Events(event registration refnum=w340, error in=w339) -> (error out=w338:errorcluster)
            n119 = call <vilib>:"Clear Errors.vi"("error in (no error)"=w338) -> ()  [unwired: 5 in, 2 out]
            n120 = call <vilib>:"Add State(s) to Queue__jki_lib_state_machine.vi"("State(s) in (\"\")"=w343) -> ("States Out"=w342:string)  [unwired: 14 in]
          }
          frame "---------- Instrument ----------" {
            n121 = Unbundle By Name(w345) -> ("SMO"=w344:refnum<class "Inst.AH2500.lvclass">)
            n122 = Bundle By Name(cluster=w345, "SMO"=w344) -> (w346:T5)
            n123 = call <vilib>:"Add State(s) to Queue__jki_lib_state_machine.vi"("State(s) in (\"\")"=w350) -> ("States Out"=w349:string)  [unwired: 14 in]
          }
          frame "Instrument: Open Hardware" {
            n124 = Unbundle By Name(w355) -> ("SMO"=w354:refnum<class "Inst.AH2500.lvclass">)
            n125 = call-dynamic "Open Hardware.vi"("error in (no error)"=w351, "Inst.AH2500 in"=w354) -> ("error out"=w352:errorcluster, "Inst.AH2500 out"=w353:refnum<class "Inst.AH2500.lvclass">)  [unwired: 8 in]
            n126 = Bundle By Name(cluster=w355, "SMO"=w353) -> (w356:T5)
            n127 = call <vilib>:"Add State(s) to Queue__jki_lib_state_machine.vi"("State(s) in (\"\")"=w359) -> ("States Out"=w358:string)  [unwired: 14 in]
          }
          frame "Instrument: Close Hardware" {
            n128 = Unbundle By Name(w364) -> ("SMO"=w363:refnum<class "Inst.AH2500.lvclass">)
            n129 = call-dynamic "Close Hardware.vi"("error in (no error)"=w360, "Inst.AH2500 in"=w363) -> ("error out"=w361:errorcluster, "Inst.AH2500 out"=w362:refnum<class "Inst.AH2500.lvclass">)  [unwired: 8 in]
            n130 = Bundle By Name(cluster=w364, "SMO"=w362) -> (w365:T5)
            n131 = call <vilib>:"Add State(s) to Queue__jki_lib_state_machine.vi"("State(s) in (\"\")"=w368) -> ("States Out"=w367:string)  [unwired: 14 in]
          }
          frame "Instrument: getAll" {
            # "communicate with\nhardware"
            n132 = Unbundle By Name(w381) -> ("SMO"=w380:refnum<class "Inst.AH2500.lvclass">)  [unwired: 2 out]
            n133 = call "Inst.AH2500.getAll.vi"("error in (no error)"=w379, "Inst.AH2500 in"=w380) -> ("error out"=w378:errorcluster, "output cluster"=w372:T9, "Inst.AH2500 out"=w377:refnum<class "Inst.AH2500.lvclass">)  [unwired: 7 in]
            n134 = call <userlib>:"setAllData.vi"("error in (no error)"=w378, "AllData"=w372, "Instrument in"=w377) -> ("error out"=w371:errorcluster, "Instrument out"=w373:refnum<class "Inst.AH2500.lvclass">)  [unwired: 7 in]
            n135 = call-dynamic "Get SMO Database Paths.vi"("error in (no error)"=w371, "Inst.AH2500 in"=w373) -> ("error out"=w370:errorcluster, "Paths"=w375:string, "Inst.AH2500 out"=w374:refnum<class "Inst.AH2500.lvclass">)  [unwired: 7 in]
            n136 = call <userlib>:"Instrument.logToDatabase.vi"("error in (no error)"=w370, "Data"=w372, "Paths"=w375, "Instrument"=w374) -> ("error out"=w369:errorcluster, "Instrument out"=w376:refnum<class "Inst.AH2500.lvclass">)  [unwired: 6 in]
            n137 = Bundle By Name(cluster=w381, "SMO"=w376) -> (w382:T5)
            n138 = call <vilib>:"Add State(s) to Queue__jki_lib_state_machine.vi"("State(s) in (\"\")"=w385) -> ("States Out"=w384:string)  [unwired: 14 in]
          }
          frame "---------- Sequence ----------" {
            n139 = call <vilib>:"Add State(s) to Queue__jki_lib_state_machine.vi"("State(s) in (\"\")"=w390) -> ("States Out"=w389:string)  [unwired: 14 in]
          }
          frame "Sequence: Status" {
            # "Sequence: Status\n(Use this frame to pass the status to the UI, this VI's UI, etc)"
            n140 = call <vilib>:"Add State(s) to Queue__jki_lib_state_machine.vi"("State(s) in (\"\")"=w396) -> ("States Out"=w395:string)  [unwired: 14 in]
            "Status" <- w391
          }
          frame "Sequence: Wait" {
            # "Sequence: Wait\n(Non-Blocking Wait)"
            # "F = repeat this state. wait\nT = go to next state. don't wait"
            n141 = Unbundle By Name(w405) -> ("Running Step"=w398:i32)
            n142 = call <userlib>:"Wait Logic.vi"("error in (no error)"=w401, "Time"=w399) -> ("error out"=w400:errorcluster, "Status String"=w397:string, "Trigger"=w402:bool)  [unwired: 6 in, 1 out]
            n143 = Increment(x=w398) -> (x+1=w412:i32)
            n144 = Select(t=w412, s=w402, f=w398) -> (s? t:f=w403:i32)
            n145 = Select(t=u32 0, s=w402, f=u32 100 ("milliseconds to wait")) -> (s? t:f=w409:u32)
            n146 = call <userlib>:"Wait (ms)__ogtk.vi"("error in (no error)"=w400, "milliseconds to wait"=w409) -> ("error out"=w407:errorcluster)  [unwired: 8 in, 1 out]
            n147 = Bundle By Name(cluster=w405, "Running Step"=w403) -> (w404:T5)
            n148 = call <vilib>:"Build State String with Arguments__JKI_lib_State_Machine.vi"("Arguments (\"\")"=w397, "State"="Sequence: Status") -> ("State with Arguments"=w406:string)  [unwired: 4 in]
            n149 = call <vilib>:"Add State(s) to Queue__jki_lib_state_machine.vi"("State(s) in Front (\"\")"=w406, "State(s) in (\"\")"=w415) -> ("States Out"=w414:string)  [unwired: 13 in]
          }
        }
      }
    }
    frame Error {
    }
  }
  n150 = call-parent "Process.vi"("error in"=w5, "Instrument"=w4) -> ("error out"=w2:errorcluster, "Instrument out"=→"Inst.AH2500 out":refnum<class "Inst.AH2500.lvclass">)  [unwired: 8 in]
  n151 = Merge Errors(w2, w1) -> (→"error out":errorcluster)
